vi "equals.vi"(8 "error in (no error)":errorcluster, 10 "Goal to Match":refnum<class "Goal.lvclass">, 11 "Goal in":refnum<class "Goal.lvclass">) -> (0 "error out":errorcluster, 2 "Equals?":bool, 3 "Goal out":refnum<class "Goal.lvclass">)   [LabVIEW 2018, in "Goal.lvclass"]
uses:
  Goal.lvclass
  Goal.lvclass/Goal.ctl
  Category/Category.lvclass
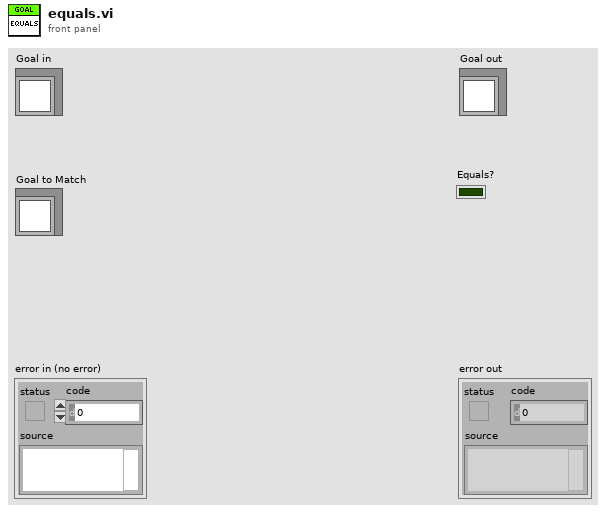
[diagram p1: front panel]
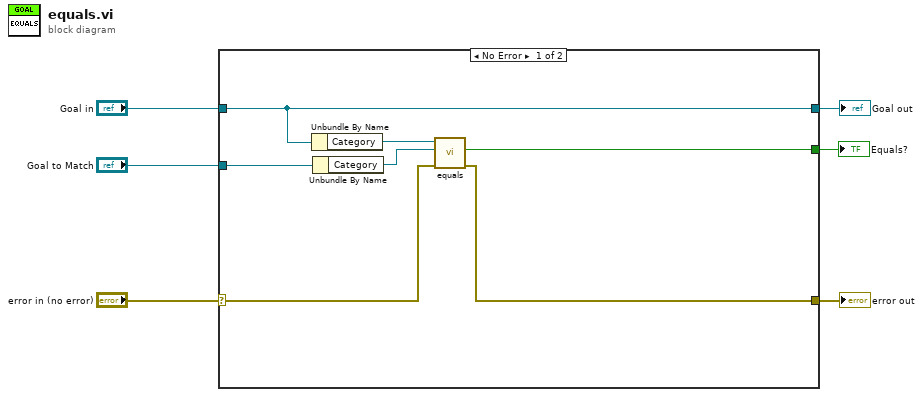
[diagram p0: block diagram]
diagram:
  n1 = case shown="No Error" "error in (no error)" {
    selector: "error in (no error)" -> [w9 w15]
    tunnel: [w8 w15] -> w5
    tunnel: [w13 w14] -> w3
    tunnel: "Goal in" -> [w13 w14]
    tunnel: "Goal to Match" -> [w12 _]
    tunnel: [w7 _] -> w1
    frame No Error {
      n2 = Unbundle By Name(w13) -> ("Category"=w11:refnum<class "Category.lvclass">)
      n3 = Unbundle By Name(w12) -> ("Category"=w10:refnum<class "Category.lvclass">)
      n4 = call "equals.vi"("error in (no error)"=w9, "Category to Match"=w10, "Category in"=w11) -> ("error out"=w8:errorcluster, "Equals?"=w7:bool)  [unwired: 6 in, 1 out]
    }
    frame Error {
    }
  }
  "error out" <- w5
  "Goal out" <- w3
  "Equals?" <- w1
